vi "Synthesize.vi"(0 "File in":refnum<class "File.lvclass">, 5 "Fs (Hz)":dbl, 7 "Npts":i32, 9 "Repetition":i32, 11 "error in (no error)":errorcluster) -> (4 "File out":refnum<class "File.lvclass">, 8 "Array":dbl[](array[numeric]), 15 "error out":errorcluster)   [LabVIEW 2020, in "File.lvclass"]
uses:
  File.lvclass
  File.lvclass/File.ctl
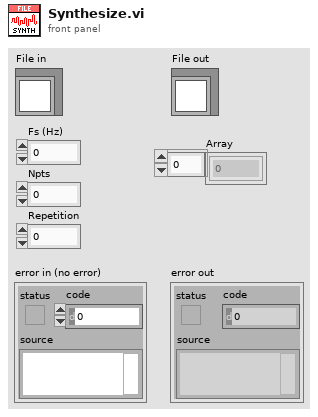
[diagram p1: front panel]
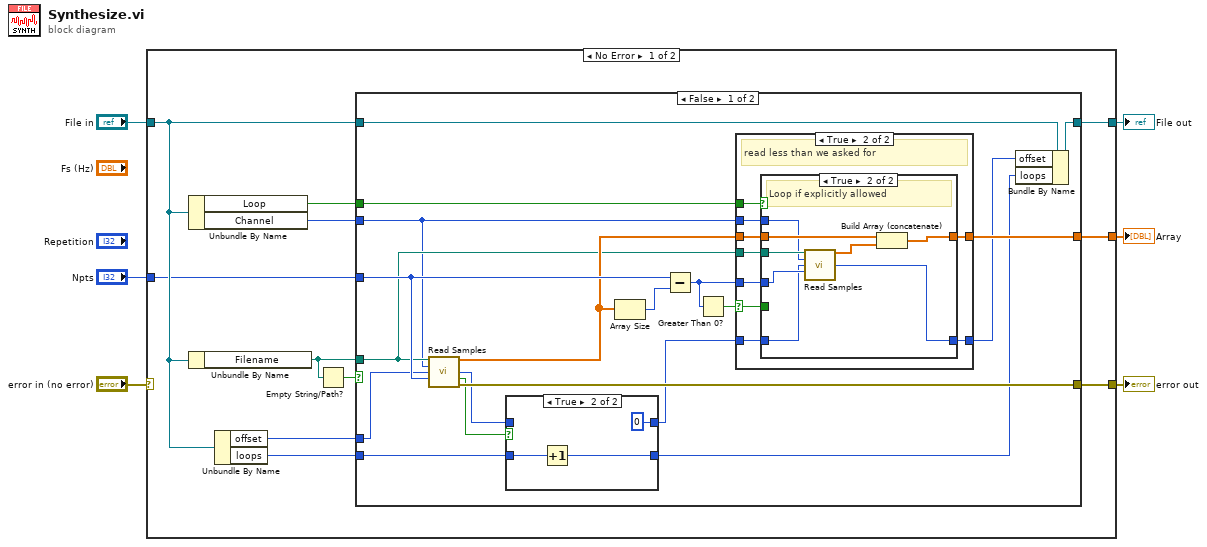
[diagram p0: block diagram]
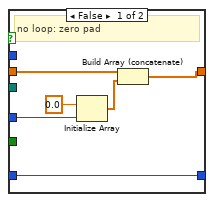
[diagram p3: hidden frame]
diagram:
  n1 = case shown="No Error" "error in (no error)" {
    selector: "error in (no error)" -> [_ w69]
    tunnel: [w8 w69] -> w6
    tunnel: [w11 w68] -> w4
    tunnel: "File in" -> [w12 w68]
    tunnel: "Npts" -> [w10 _]
    tunnel: [w9 _] -> w1
    frame No Error {
      n2 = Unbundle By Name(w12) -> ("Loop"=w7:bool, "Channel"=w15:i32)
      n3 = Unbundle By Name(w12) -> ("Filename"=w14:path)
      n4 = Unbundle By Name(w12) -> ("offset"=w16:i32, "loops"=w17:i32)
      n5 = Empty String/Path?(string/path=w14) -> (empty?=w13:bool)
      n6 = case shown="False" w13 {
        tunnel: w14 -> [w19 _]
        tunnel: [w36 _] -> w8
        tunnel: w10 -> [w29 _]
        tunnel: w15 -> [w18 _]
        tunnel: w16 -> [w23 _]
        tunnel: w12 -> [w32 w67]
        tunnel: [w31 w67] -> w11
        tunnel: [w30 _] -> w9
        tunnel: w17 -> [w27 _]
        tunnel: w7 -> [w22 _]
        frame False {
          n7 = call "Read Samples.vi"("Filename"=w19, "channel"=w18, "offset in"=w23, "Npts"=w29) -> ("Samples"=w28:dbl[], "offset out"=w25:i32, "end of file?"=w26:bool, "error out"=w36:errorcluster)  [unwired: 8 in]
          n8 = case shown="True" w26 {
            tunnel: w27 -> [w63 w65]
            tunnel: w25 -> [w62 _]
            tunnel: [w62 0] -> w21
            tunnel: [w63 w64] -> w24
            frame False {
            }
            frame True {
              n9 = Increment(x=w65) -> (x+1=w64:i32)
            }
          }
          n10 = Array Size(array=w28) -> (size(s)=w35:i32)
          n11 = Subtract(x=w29, y=w35) -> (x-y=w33:i32)
          n12 = Greater Than 0?(x=w33) -> (x > 0?=w34:bool)
          n13 = case shown="True" w34 {
            selector: w34 -> [_ w47]
            tunnel: w33 -> [_ w46]
            tunnel: [w38 w45] -> w30
            tunnel: w28 -> [w38 w44]
            tunnel: w22 -> [_ w43]
            tunnel: w21 -> [w37 w42]
            tunnel: [w37 w41] -> w20
            tunnel: w19 -> [_ w40]
            tunnel: w18 -> [_ w39]
            frame False {
              # "got what we asked for, all good"
            }
            frame True {
              # "read less than we asked for"
              n14 = case shown="True" w43 {
                tunnel: w44 -> [w53 w61]
                tunnel: w46 -> [w50 w58]
                tunnel: [w52 w56] -> w45
                tunnel: w47 -> [_ _]
                tunnel: w42 -> [w48 w57]
                tunnel: [w48 w54] -> w41
                tunnel: w40 -> [_ w60]
                tunnel: w39 -> [_ w59]
                frame False {
                  # "no loop: zero pad"
                  n15 = Initialize Array(0.0 ("element"), w50) -> (w51:dbl[])
                  n16 = Build Array (concatenate)(w53, w51) -> (w52:dbl[])
                }
                frame True {
                  # "Loop if explicitly allowed"
                  n17 = call "Read Samples.vi"("Filename"=w60, "channel"=w59, "offset in"=w57, "Npts"=w58) -> ("Samples"=w55:dbl[], "offset out"=w54:i32)  [unwired: 8 in, 2 out]
                  n18 = Build Array (concatenate)(w61, w55) -> (w56:dbl[])
                }
              }
            }
          }
          n19 = Bundle By Name(cluster=w32, "offset"=w20, "loops"=w24) -> (w31:refnum<class "File.lvclass">)
        }
        frame True {
        }
      }
    }
    frame Error {
    }
  }
  "error out" <- w6
  "File out" <- w4
  "Array" <- w1
